vi "WriteU64ToU8FIFO.vi"(1 "FIFO":refnum<k21>, 2 "Value":u64) -> (0 "FIFO":refnum<k21>)   [LabVIEW 2023]
uses:
  <vilib>/rvi/DataTransferAndStorage/Container/Common/niFpgaContainerExecOnDevCompGetState.vi
  <vilib>/rvi/Emulation/niFpgaEmulationIsFPGAContextNoSignature.vi
  <vilib>/rvi/Emulation/niFpgaSctlEmulationGetInTimedLoop.vi
  <vilib>/rvi/errors/niFpgaSetErrorForExecOnDevCompSimple.vi
  <vilib>/rvi/eio/common/nirviEmuReportErrorAndStop.vi
  <vilib>/rvi/DataTransferAndStorage/Container/Common/niFpgaContainerGetUniqueNameForEmu.vi
  <vilib>/rvi/FIFO/Fifo_Resource/nirvififoEmulationSetSize.vi
  <vilib>/rvi/FIFO/Fifo_Resource/nirviFifoEmulationQueueMgr.vi
  <instcachedir>/0/nirviFifoEmulationQueueMgr_E5CAEC123FF24DC58D834DCA3CDAA9B5.lvgen/nirviFifoEmulationQueueMgr_E5CAEC123FF24DC58D834DCA3CDAA9B5_002.vi
  <vilib>/rvi/FIFO/Fifo_Resource/nirvififoEmulationDetermineInputValidOut.vi
  <vilib>/rvi/FIFO/Fifo_Resource/nirvififoEmulationCreateLock.vi
  <vilib>/rvi/Emulation/niFpgaProcessEmulError.vi
  <vilib>/rvi/FIFO/Fifo_Resource/nirvififoEmulationObtainLock.vi
  <vilib>/rvi/FIFO/Fifo_Resource/nirvififoEmulationReleaseLock.vi
  <vilib>/rvi/occurrence/nirviWaitOnOccurrenceBase.vi
  <vilib>/rvi/errors/nirviReportUnexpectedCaseInternalError.vi
  <vilib>/rvi/errors/nirviReportUnexpectedCaseInternalError (U32).vi
  <vilib>/Utility/error.llb/Clear Errors.vi
  <vilib>/eio/utilities/niEioResolveVilibRelativePath.vi
  <vilib>/rvi/interface/RandomDataEmulation/niFpgaRandomDataHandleErrors.vi
  <vilib>/rvi/DataTransferAndStorage/Container/XNode/niFpgaContainer.xnode
  <vilib>/rvi/FIFO/Fifo_Resource/niFpgaFifoEmulationRefIn.vi
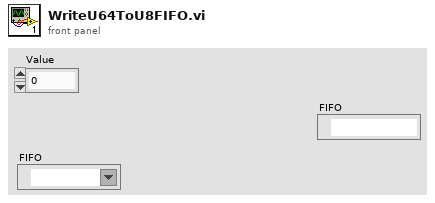
[diagram p1: front panel]
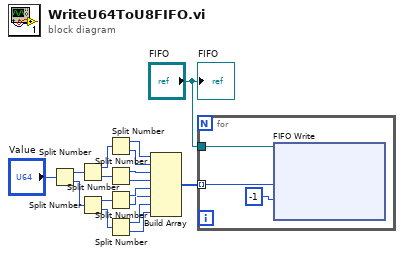
[diagram p0: block diagram]
diagram:
  n1 = Split Number(x="Value") -> (hi(x)=w16:u32, lo(x)=w15:u32)
  n2 = Split Number(x=w16) -> (hi(x)=w14:u16, lo(x)=w13:u16)
  n3 = Split Number(x=w15) -> (hi(x)=w12:u16, lo(x)=w11:u16)
  n4 = Split Number(x=w14) -> (hi(x)=w10:u8, lo(x)=w9:u8)
  n5 = Split Number(x=w13) -> (hi(x)=w8:u8, lo(x)=w7:u8)
  n6 = Split Number(x=w12) -> (hi(x)=w6:u8, lo(x)=w5:u8)
  n7 = Split Number(x=w11) -> (hi(x)=w4:u8, lo(x)=w3:u8)
  n8 = Build Array(w10, w9, w8, w7, w6, w5, w4, w3) -> (w2:u8[])
  n9 = for {
    tunnel: "FIFO" -> [w20]
    tunnel: w2 -> [w19] mode=indexing
    n10 = xnode "FIFO Write"("Element"=w19, "Timeout"=-1, "FIFO In"=w20) -> ()  [unwired: 2 out]
  }
  "FIFO" <- "FIFO"
